vi "Moving_Point_Average.vi"(10 "Averaging Points":i32, 11 "X":dbl[](array[numeric])) -> (0 "Actual Averaging":i32, 2 "Moving Average of X":dbl[](array[numeric]))   [LabVIEW 2022 SP3]
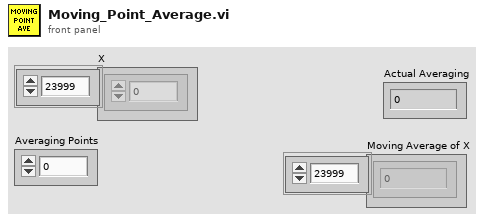
[diagram p1: front panel]
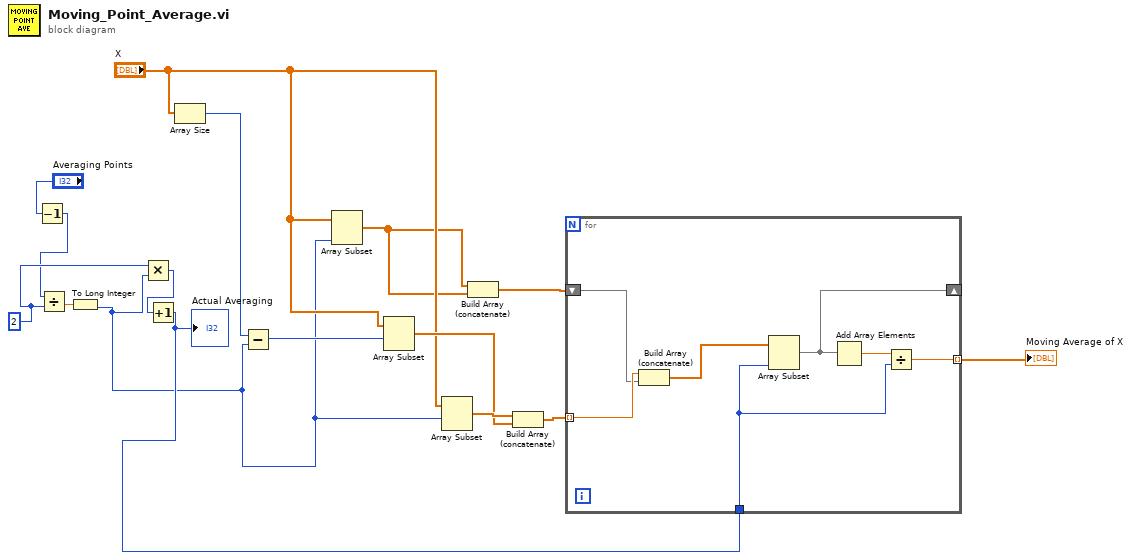
[diagram p0: block diagram]
diagram:
  w5 = 2 ("y")
  n1 = Decrement(x="Averaging Points") -> (x-1=w2:i32)
  n2 = Divide(x=w2, y=w5) -> (x/y=w8:dbl)
  n3 = To Long Integer(number=w8) -> (32bit integer=w6:i32)
  n4 = Multiply(x=w5, y=w6) -> (x*y=w4:i32)
  n5 = Increment(x=w4) -> (x+1=w7:i32)
  "Actual Averaging" <- w7
  n6 = Array Size(array="X") -> (size(s)=w10:i32)
  n7 = Subtract(x=w10, y=w6) -> (x-y=w13:i32)
  n8 = Array Subset(array="X", length=w6) -> (w1:dbl[])  [unwired: 1 in]
  n9 = Array Subset(array="X", index=w13) -> (w15:dbl[])  [unwired: 1 in]
  n10 = Array Subset(array="X", index=w6) -> (w16:dbl[])  [unwired: 1 in]
  n11 = Build Array (concatenate)(w1, w1) -> (w12:dbl[])
  n12 = Build Array (concatenate)(w16, w15) -> (w14:dbl[])
  n13 = for {
    shift-right: [w18] -> _
    shift-left: w12 -> [w22]
    tunnel: w14 -> [w23] mode=indexing
    tunnel: w7 -> [w19]
    tunnel: [w17] -> w9 mode=indexing
    n14 = Build Array (concatenate)(w23, w22) -> (w21:dbl[])
    n15 = Array Subset(array=w21, length=w19) -> (w18:dbl[])  [unwired: 1 in]
    n16 = Add Array Elements(numeric array=w18) -> (sum=w20:dbl)
    n17 = Divide(x=w20, y=w19) -> (x/y=w17:dbl)
  }
  "Moving Average of X" <- w9
